vi "Engine(CSM).vi"(7 "Name(\"\" to use uuid)":string="TSEngine") -> ()   [LabVIEW 2020, in "CSMStand(Lite).lvlib"]
doc: "------------- lvcsm -------------\n[CSMStates]\nItem 0 = \"Idle\"\nItem 1 = \"CSM Documentation\"\nItem 2 = \"Error Handler\"\nItem 3 = \"VI Reference\"\nItem 4 = \"Critical Error\"\nItem 5 = \"Target Timeout Error\"\nItem 6 = \"Target Error\"\nItem 7 = \"Async Response\"\nItem 8 = \"Response\"\nItem 9 = \"Async Message Posted\"\nItem 10 = \"Initialize Core Data\"\nItem 11 = \"Exit\"\nItem 12 = \"Data: Initialize\"\nItem 13 = \"Data: Get Configuration\"\nItem 14 = \"Data: Get Internal Data\"\nItem 15 = \"Data: Set Configuration\"\nItem 16 = \"Data: Update Indicators\"\nItem 17 = \"Data: Cleanup\"\nItem 18 = \"Macro: Initialize\"\nItem 19 = \"Macro: Exit\"\nItem 20 = \"TS: Load Sequence\"\nItem 21 = \"TS: Unload Sequence\"\nItem 22 = \"TS: SinglePass\"\nItem 23 = \"TS: Terminate\"\n\n[CSMStatus]\nItem 0 = \"Error Occurred@Error Handler\"\nItem 1 = \"SequenceLoaded Event@TS: Load Sequence\"\nItem 2 = \"SequenceUnloaded Event@TS: Unload Sequence\""
uses:
  CSMStand(Lite).lvlib
  177df613-786b-4953-91e1-5a54b4498db6.vi
  e32ef8e6-06f2-447d-b550-f32965c6f747.vi
  42464f7e-1352-40b0-9025-febecf2bff56.vi
  28b741bb-94bb-4c2f-9535-6203235cad54.vi
  67be72c3-d4c2-4166-a53e-31f1adb5f8f9.vi
  <userlib>/_NEVSTOP/Communicable State Machine(CSM)/_Support/Common/Format Timestamp.vi
  <userlib>/_NEVSTOP/Communicable State Machine(CSM)/AdvanceAPI/CSM - Make String Arguments Safe.vi
  <userlib>/_NEVSTOP/Communicable State Machine(CSM)/AdvanceAPI/CSM - Break Down Multiple States String.vi
  <userlib>/_NEVSTOP/Communicable State Machine(CSM)/AdvanceAPI/CSM - Compact Multiple States.vi
  <userlib>/_NEVSTOP/Communicable State Machine(CSM)/AdvanceAPI/CSM - Keywords.vi
  <userlib>/_NEVSTOP/Communicable State Machine(CSM)/_Shared/Trim Single-line Text.vi
  <userlib>/_NEVSTOP/Communicable State Machine(CSM)/addons/API-String-Arugments-Support/_Support/Query Data as API String Arguments(variant).vi
  <userlib>/_NEVSTOP/Communicable State Machine(CSM)/addons/API-String-Arugments-Support/_Support/Convert API String Arguments to Data(variant).vi
  _Support/Working Thread.vi
  <userlib>/_NEVSTOP/Communicable State Machine(CSM)/AdvanceAPI/CSM - Get Module Attribute.vi
  <userlib>/_NEVSTOP/Communicable State Machine(CSM)/AdvanceAPI/CSM - Set Module Attribute.vi
  <userlib>/_NEVSTOP/Communicable State Machine(CSM)/Communicable State Machine.lvlib
  <userlib>/_NEVSTOP/Communicable State Machine(CSM)/addons/API-String-Arugments-Support/API String Arguments Support.lvlib
panel:
  out "State History":string
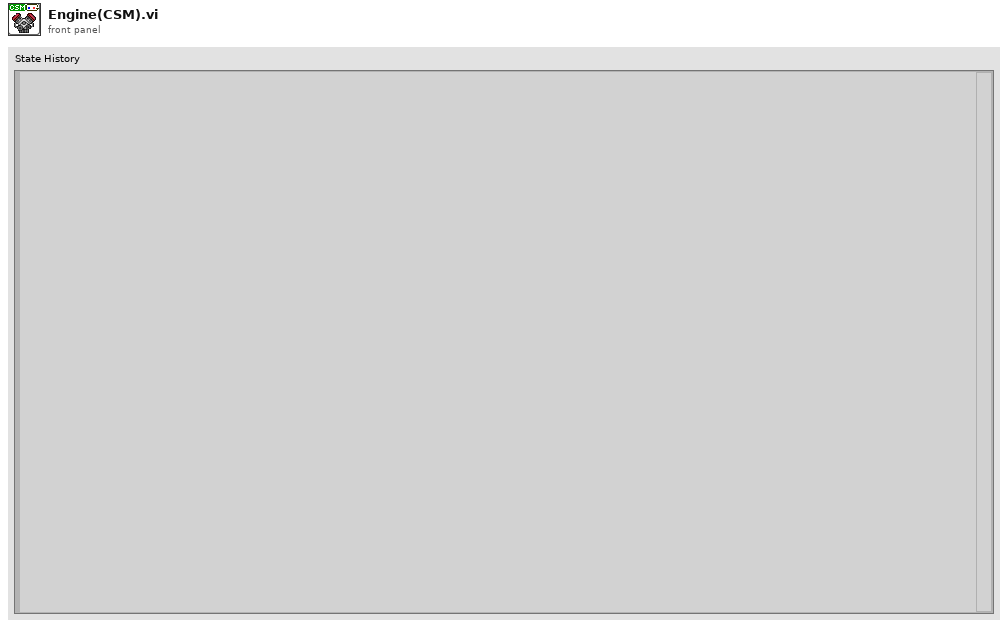
[diagram p1: front panel]
types:
  T1 = enum32{"Invalid", "Standard", "Closed", "Hidden", "Minimized", "Maximized"}
  T2 = enum32{"invalid app kind", "Development System", "Run Time System", "Student Edition", "Embedded LabVIEW", "Evaluation", "Custom"}
  T3 = typedef "Communicable State Machine.lvlib/_CSM_Response Source Message.ctl" = cluster{"‘State":string, "’Arguments":string, "’Error":errorcluster}
  T4 = cluster{"Current VI Reference":refnum<vi>, "Close Panel on Exit?":bool}
  T5 = cluster{"Core":cluster{"Current VI Reference":refnum<vi>, "Close Panel on Exit?":bool}, "Sequence":string}
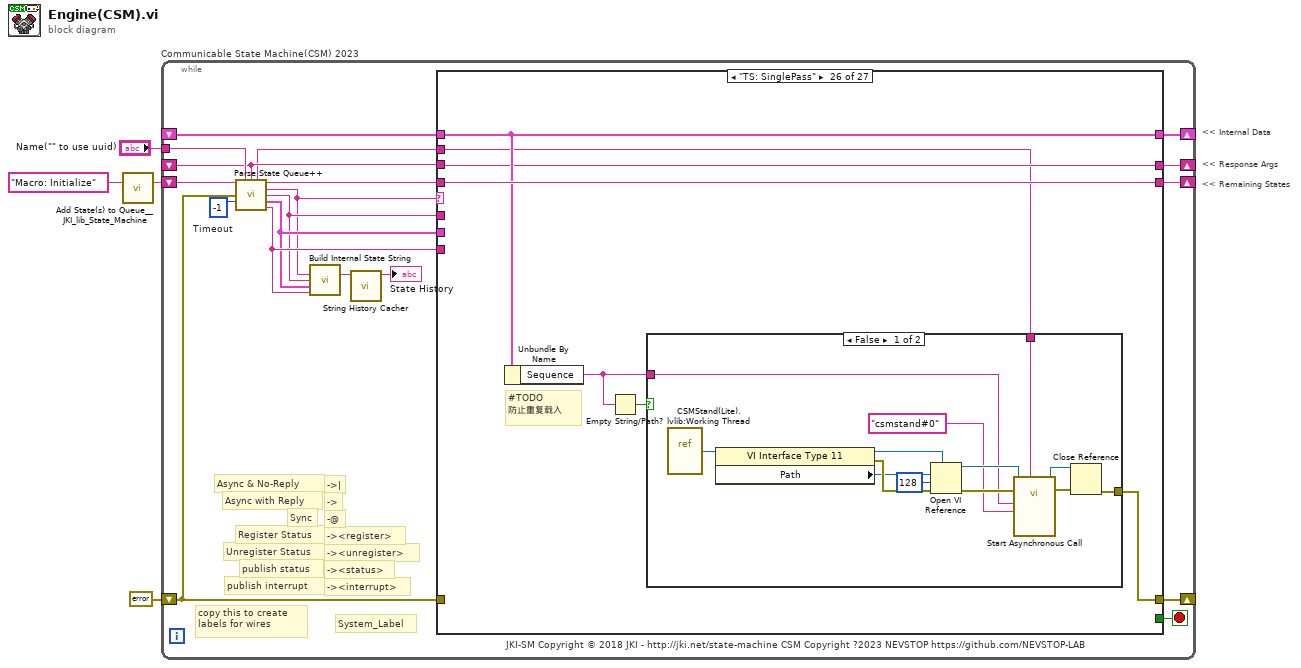
[diagram p0: block diagram]
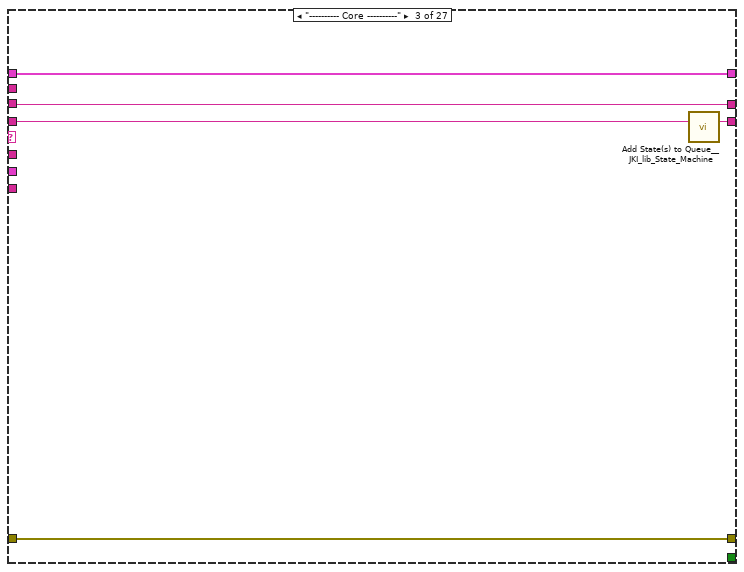
[diagram p4: hidden frame]
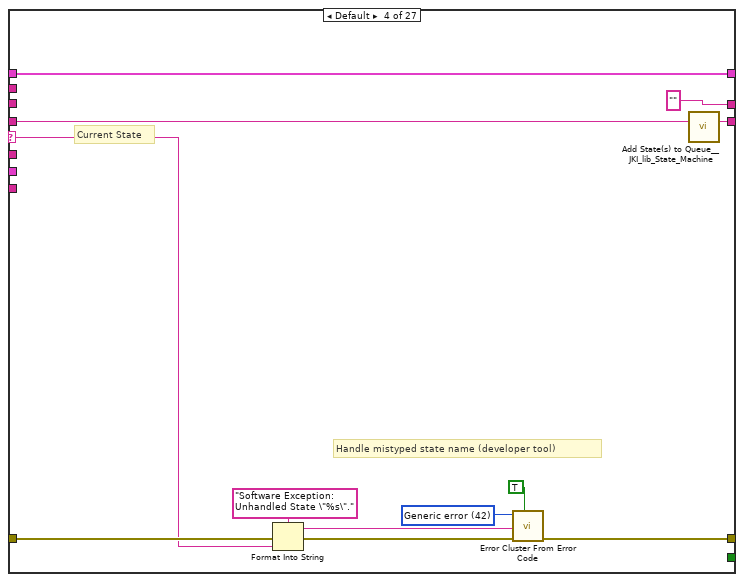
[diagram p5: hidden frame]
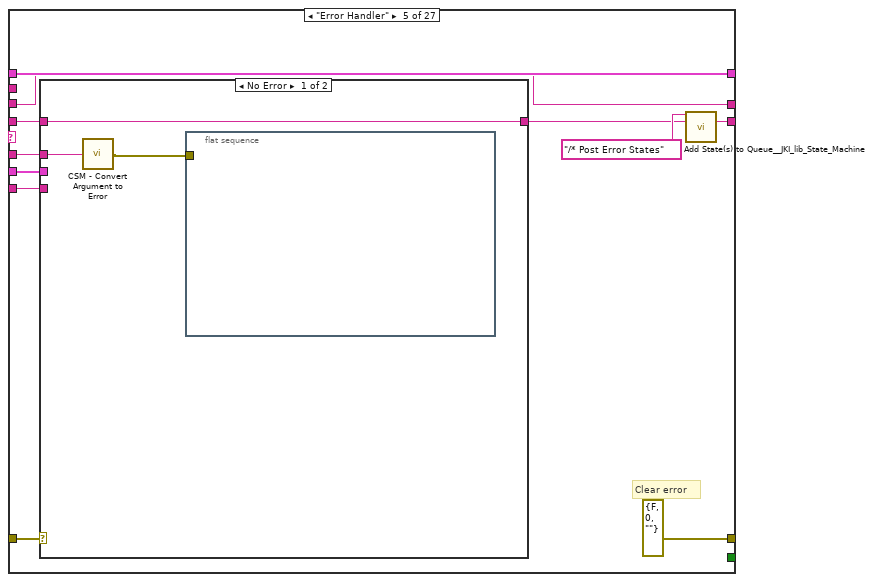
[diagram p6: hidden frame]
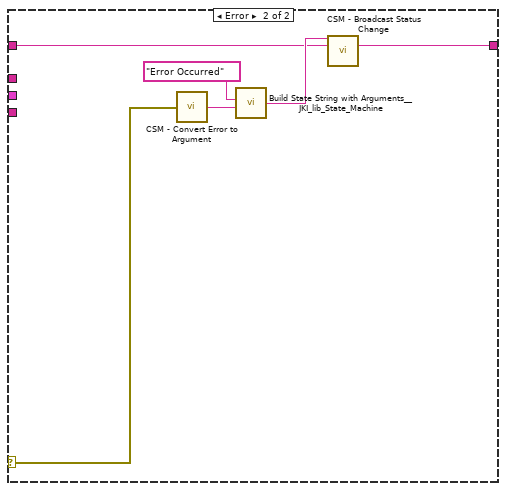
[diagram p7: hidden frame]
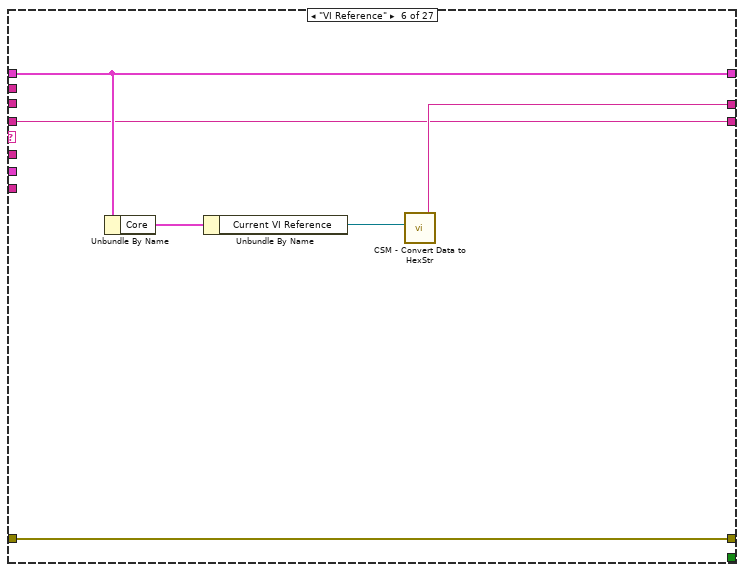
[diagram p8: hidden frame]
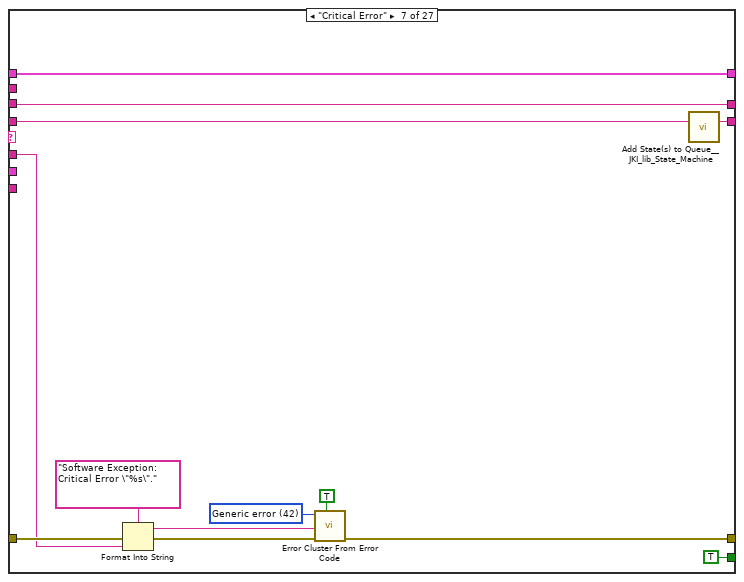
[diagram p9: hidden frame]
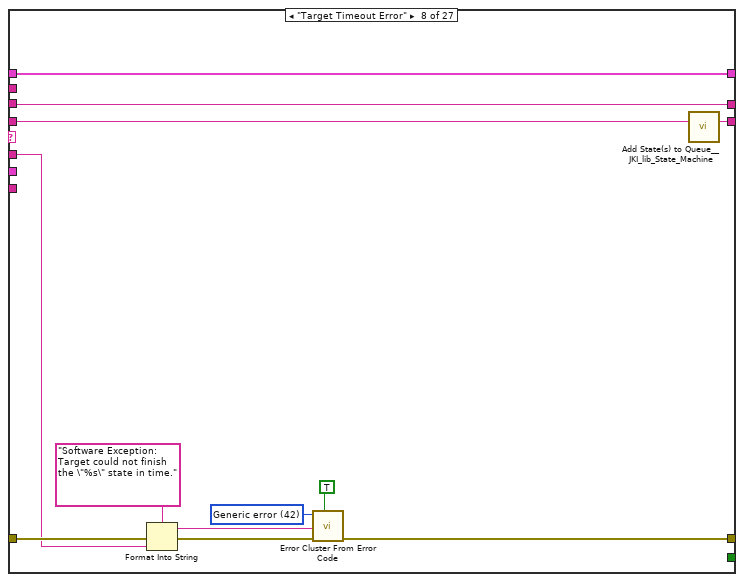
[diagram p10: hidden frame]
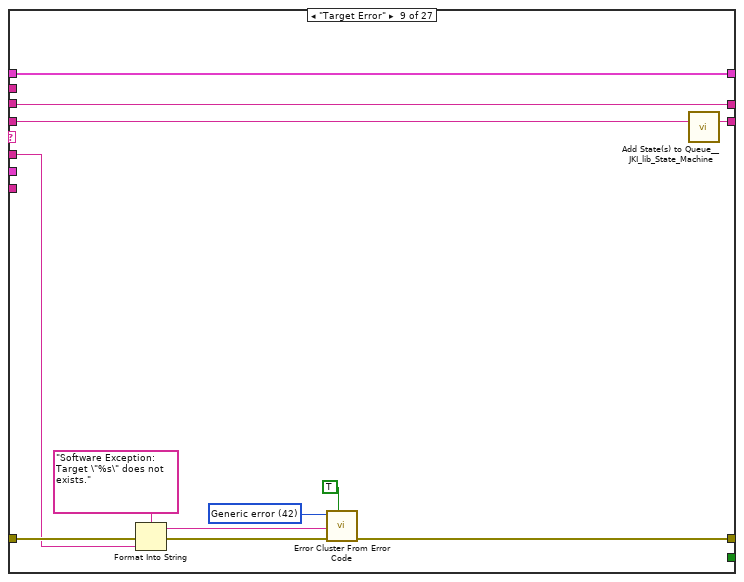
[diagram p11: hidden frame]
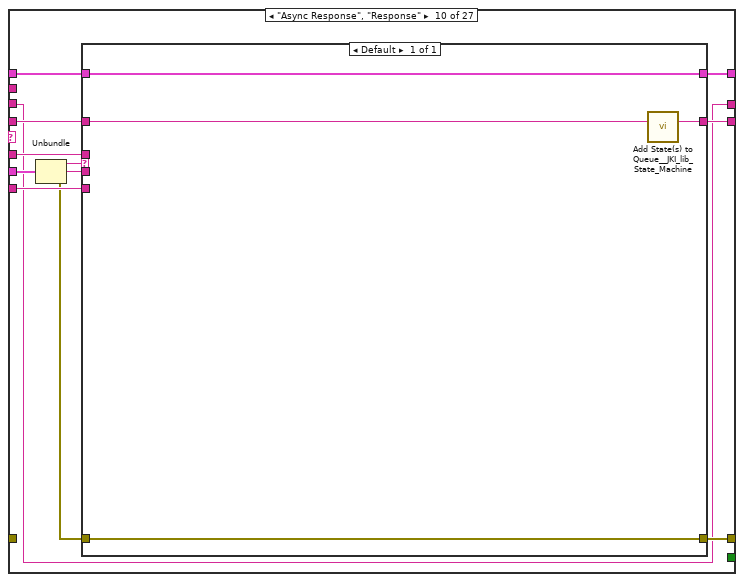
[diagram p12: hidden frame]
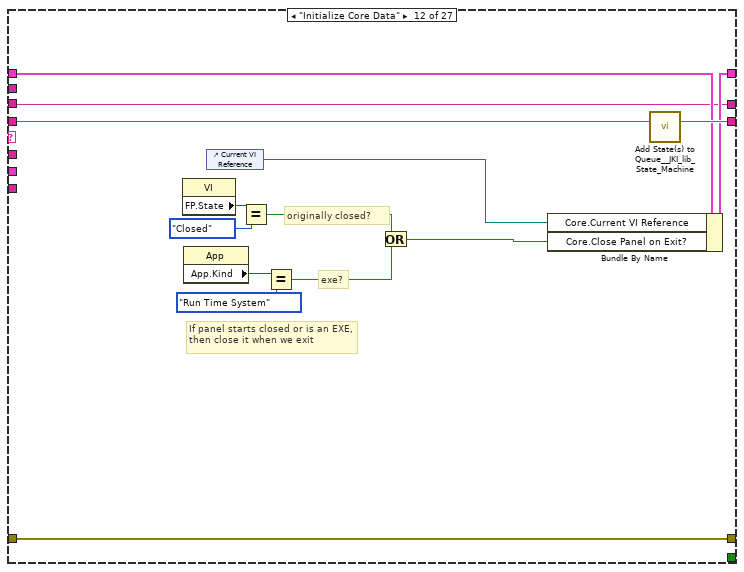
[diagram p14: hidden frame]
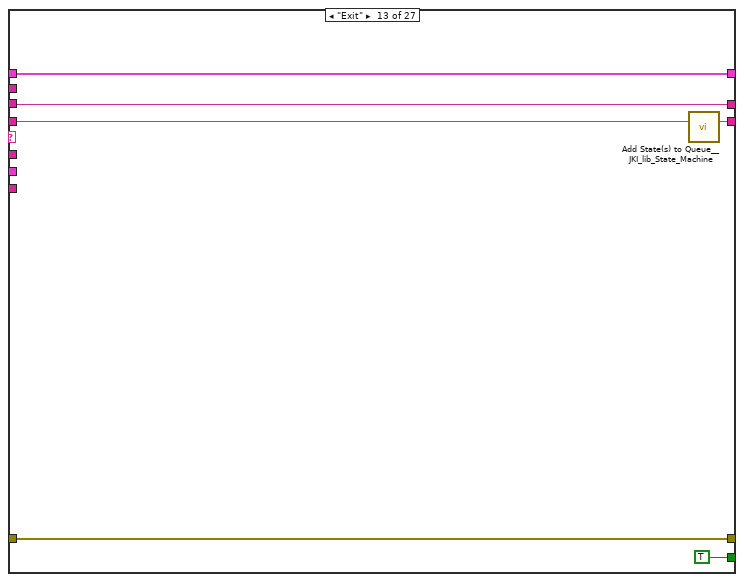
[diagram p15: hidden frame]
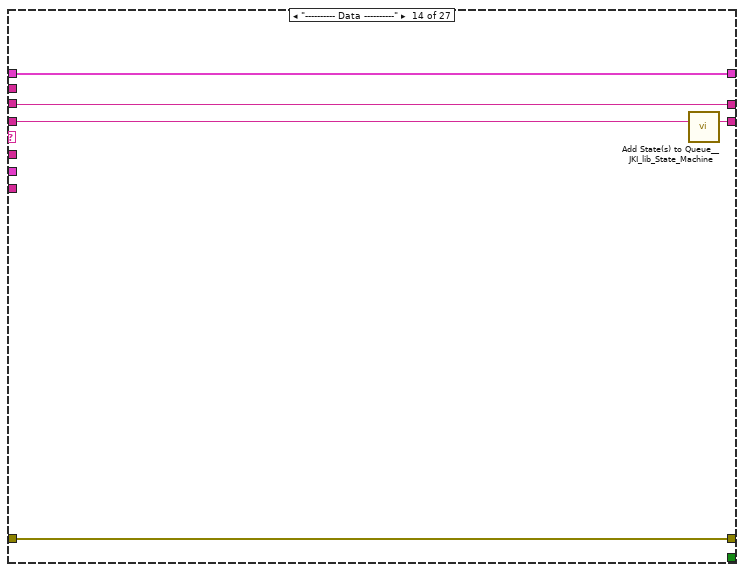
[diagram p16: hidden frame]
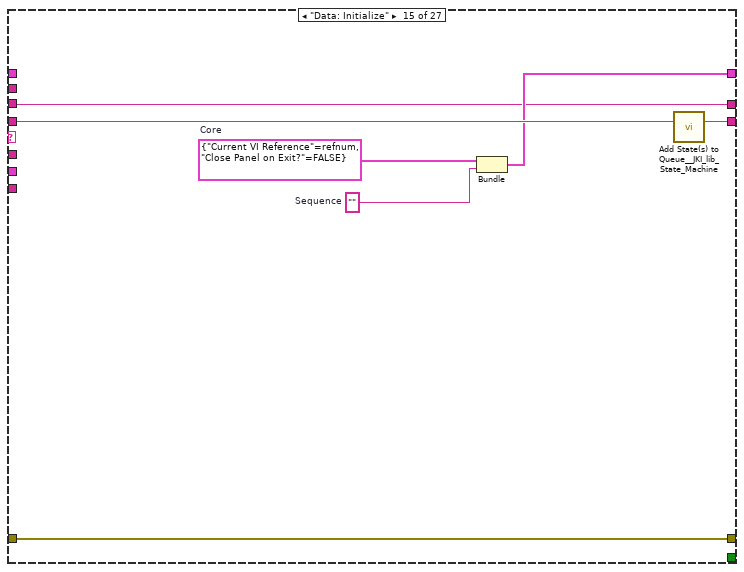
[diagram p17: hidden frame]
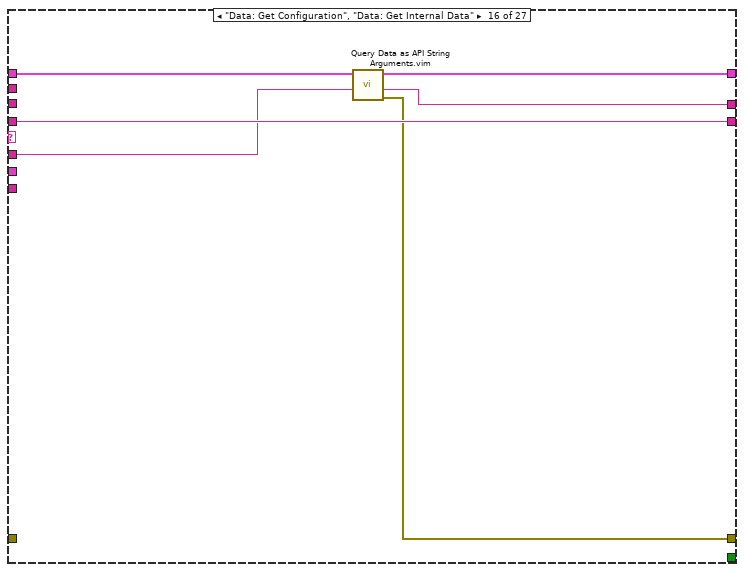
[diagram p18: hidden frame]
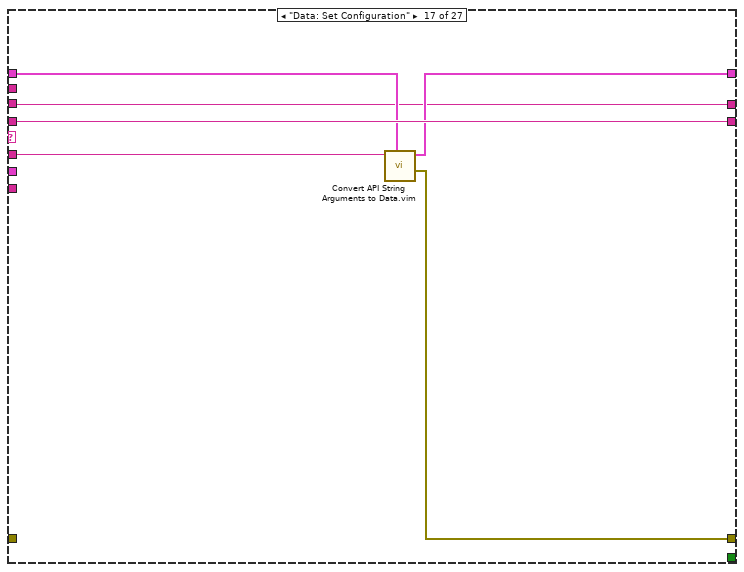
[diagram p19: hidden frame]
diagram:
  # "<< Internal Data"
  # "<< Response Args"
  # "<< Remaining States"
  n1 = call <vilib>:"Add State(s) to Queue__JKI_lib_State_Machine.vi"("State(s) in (\"\")"="Macro: Initialize" ("Init States(\"Macro: Initialize\")")) -> ("States Out"=w3:string)  [unwired: 14 in]
  n2 = while "Communicable State Machine(CSM) 2023" {
    shift-right: [w18] -> _
    shift-left: _ -> [w17]
    shift-right: [w21] -> _
    shift-left: errorcluster {"status"=FALSE, "code"=0, "source"=""} ("error out") -> [w5]
    shift-right: [w20] -> _
    shift-left: w3 -> [w22]
    tunnel: "Name(\"\" to use uuid)" -> [w14]
    shift-right: [w15] -> _
    shift-left: _ -> [w7]
    stop <- w19 stop-if-true
    w16 = -1  # Timeout
    # "copy this to create labels for wires"
    # "System_Label"
    # "-><interrupt>"
    # "-><status>"
    # "-><unregister>"
    # "-><register>"
    # "-@"
    # "->"
    # "->|"
    # "publish interrupt"
    # "publish status"
    # "Unregister Status"
    # "Register Status"
    # "Sync"
    # "Async with Reply"
    # "Async & No-Reply"
    # "JKI-SM Copyright © 2018 JKI - http://jki.net/state-machine CSM Copyright ?2023 NEVSTOP https://github.com/NEVSTOP-LAB"
    n3 = call <userlib>:"Parse State Queue++.vi"("State Queue"=w22, "Name (\"\" to Use UUID)"=w14, "Response Arguments"=w7, "Previous Error"=w5, "Dequeue (1 ms)"=w16) -> ("Name Used"=w6:string, "Remaining States"=w23:string, "Current State"=w8:string, "Arguments"=w9:string, ">> Response Source Message >>"=w10:T3, ">> Source CSM >>"=w11:string)  [unwired: 5 in]
    n4 = call <userlib>:"Build Internal State String.vi"("State"=w8, "Arguments (\"\")"=w9, ">> Response Source Message >>"=w10, "Source (\"\")"=w11) -> ("State With Arguments"=w12:string)  [unwired: 11 in]
    n5 = call <userlib>:"String History Cacher.vi"("String"=w12) -> ("String Cache"=→"State History":string)  [unwired: 10 in]
    n6 = case shown="\"TS: SinglePass\"" w8 {
      selector: w8 -> [_ _ _ w38 _ _ _ _ _ _ _ _ _ _ _ _ _ _ _ _ _ _ _ _ _ _ _]
      tunnel: w23 -> [w25 w30 w36 w42 w53 w70 w81 w94 w106 w117 w130 w145 w151 w156 w163 w169 w175 w178 w186 w191 w197 w203 w206 w213 w220 w230 w259]
      tunnel: w9 -> [_ _ _ _ w52 _ w77 w90 w102 w116 _ _ _ _ _ w164 w174 _ _ _ _ _ _ w209 _ _ w257]
      tunnel: w17 -> [w26 w29 w33 w40 w58 w74 w79 w92 w104 w118 w129 w138 w149 w153 _ w168 w173 w177 w181 w188 w194 w200 w205 w216 w222 w229 w258]
      tunnel: [w27 w31 w34 w44 errorcluster {"status"=FALSE, "code"=0, "source"=""} ("error out") w69 w83 w89 w101 w121 w131 w142 w148 w154 w160 w165 w171 w179 w182 w189 w195 w201 w207 w217 w223 w228 w251] -> w21
      tunnel: w5 -> [w27 w31 w34 w43 w56 w69 w82 w95 w107 _ w131 w142 w148 w154 w160 _ _ w179 w183 w189 w195 w201 w207 w217 w223 _ _]
      tunnel: [w25 w30 w35 w41 w54 w70 w80 w93 w105 w119 w130 w144 w150 w155 w162 w169 w175 w178 w185 w190 w196 w202 w206 w214 w221 w230 w259] -> w20
      tunnel: [_ _ _ _ _ _ TRUE _ _ _ _ _ TRUE _ _ _ _ _ _ _ _ _ _ _ _ _ _] -> w19
      tunnel: [w26 w29 w33 w40 w58 w74 w79 w92 w104 w120 w129 w143 w149 w153 w161 w167 w172 w177 w181 w188 w194 w200 w205 w215 w222 w229 w258] -> w18
      tunnel: w11 -> [_ _ _ _ w51 _ _ _ _ w114 _ _ _ _ _ _ _ _ _ _ _ _ _ _ _ _ _]
      tunnel: w10 -> [_ _ _ _ w50 _ _ _ _ w115 _ _ _ _ _ _ _ _ _ _ _ _ _ _ _ _ _]
      tunnel: [w24 w28 w32 "" w49 w71 w75 w88 w100 w112 w128 w132 w146 w152 w157 w166 w170 w176 w180 w187 w192 w198 w204 w208 w218 w227 w253] -> w15
      tunnel: w6 -> [_ _ _ _ _ _ _ _ _ _ _ _ _ _ _ _ _ _ _ _ _ _ _ _ _ w226 w247]
      tunnel: w7 -> [w24 w28 w32 _ w49 _ w75 w88 w100 w112 w128 w132 w146 w152 w157 _ w170 w176 w180 w187 w192 w198 w204 w208 w218 w227 w253]
      frame "", "Idle" {
      }
      frame "CSM Documentation" {
      }
      frame "---------- Core ----------" {
        n7 = call <vilib>:"Add State(s) to Queue__JKI_lib_State_Machine.vi"("State(s) in (\"\")"=w36) -> ("States Out"=w35:string)  [unwired: 14 in]
      }
      frame Default {
        w47 = 42 items=["No error", "Argument error", "Memory is full", "Out of zone", "End of file", "File already open", "Generic file I/O error", "File not found", "File permission error", "Disk is full", "Duplicate path", "Too many files open", "System feature not enabled", "Resource file not found", "Cannot add resource", "Resource not found", "Image not found", "Image memory error", "Pen does not exist", "Config type invalid", "Config token not found", "Config parse error", "Config memory error", "Bad external code format", "Bad external code offset", "External code not present", "Null window", "Destroy window error", "Null menu", "Print aborted", "Bad print record", "Print driver error", "Windows error during printing", "Memory error during printing", "Print dialog error", "Generic print error", "Invalid device refnum", "Device not found", "Device parameter error", "Device unit error", "Cannot open device", "Device call aborted", "Generic error", "Cancelled by user", "Object ID too low", "Object ID too high", "Object not in heap", "Unknown heap", "Unknown object (invalid DefProc)", "Unknown object (DefProc not in table)", "Message out of range", "Invalid (null) method", "Unknown message", "Manager call not supported", "Bad address", "Network operation in progress", "Network operation timed out", "Connection is busy", "Network attribute not supported", "Network error", "Address in use", "System out of memory", "Connection aborted", "Connection refused", "Not connected", "Already connected", "Connection closed", "Initialization error (interapplication manager)", "Bad occurrence", "Wait on unbound occurrence handler", "Occurrence queue overflow", "Datalog type conflict", "Unused", "Unrecognized type (interapplication manager)", "Memory corrupt", "Failed to make temporary DLL", "Old CIN version", "Drag socket not found", "Failed to load drop-object", "Failed to register OLE object", "Failed to release OLE object", "Format specifier type mismatch", "Unknown format specifier", "Too few format specifiers", "Too many format specifiers", "Scan failed", "Newer CIN version", "Error converting to variant", "Runtime menu error", "Password tampered", "Variant attribute not found", "Incompatible variant data type", "Event data is not available", "Event Store is not present", "Occurrence is not found", "Event Queue is not created", "Event info is not available", "Refnum passed is NULL", "Error retrieving Class GUID", "Error retrieving CoClass GUID", "Error retrieving TypeLib GUID.", "Bad built application magic bytes.", "Specific driver is different from the specific driver associated with the Logical Name.", "There is no session opened to the class driver.", "Max Error", "MAX - Error with config objects", "MAX - Error loading configuration", "MAX - Group not supported"]
        # "Current State"
        # "Handle mistyped state name (developer tool)"
        n8 = Format Into String(format string="Software Exception: Unhandled State \"%s\"." ("message"), error in=w43, w38) -> (resulting string=w46:string, error out=w45:errorcluster)  [unwired: 1 in]
        n9 = call <vilib>:"Error Cluster From Error Code.vi"("show call chain? (False)"=TRUE, "error in (no error)"=w45, "error message (\"\")"=w46, "error code (0)"=w47) -> ("error out"=w44:errorcluster)  [unwired: 5 in]
        n10 = call <vilib>:"Add State(s) to Queue__JKI_lib_State_Machine.vi"("State(s) in (\"\")"=w42) -> ("States Out"=w41:string)  [unwired: 14 in]
      }
      frame "Error Handler" {
        # "Clear error"
        n11 = case shown="No Error" w56 {
          selector: w56 -> [_ w63]
          tunnel: [w62 w65] -> w55
          tunnel: w53 -> [w62 w64]
          tunnel: w52 -> [w61 _]
          tunnel: w51 -> [_ _]
          tunnel: w50 -> [_ _]
          frame No Error {
            n12 = call <userlib>:"CSM - Convert Argument to Error.vi"("Argument"=w61) -> ("Error"=w60:errorcluster)  [unwired: 4 in]
            n13 = flat-sequence {
              tunnel: w60 -> [_]
              frame #0 {
              }
            }
          }
          frame Error {
            n14 = call <userlib>:"CSM - Convert Error to Argument.vi"("Error"=w63) -> ("Argument"=w67:string)  [unwired: 4 in]
            n15 = call <vilib>:"Build State String with Arguments__JKI_lib_State_Machine.vi"("Arguments (\"\")"=w67, "State"="Error Occurred" ("Status with Arguments")) -> ("State with Arguments"=w66:string)  [unwired: 4 in]
            n16 = call <userlib>:"CSM - Broadcast Status Change.vi"("Status With Arguments"=w66, "State Queue"=w64) -> ("Remaining States"=w65:string)  [unwired: 13 in]
          }
        }
        n17 = call <vilib>:"Add State(s) to Queue__JKI_lib_State_Machine.vi"("State(s) in Front (\"\")"="/* Post Error States", "State(s) in (\"\")"=w55) -> ("States Out"=w54:string)  [unwired: 13 in]
      }
      frame "VI Reference" {
        n18 = Unbundle By Name(w74) -> ("Core"=w73:T4)
        n19 = Unbundle By Name(w73) -> ("Current VI Reference"=w72:refnum<vi>)
        n20 = call <userlib>:"CSM - Convert Data to HexStr.vi"("Variant"=w72) -> ("HEX String (0-9,A-F)"=w71:string)  [unwired: 8 in]
      }
      frame "Critical Error" {
        w86 = 42 items=["No error", "Argument error", "Memory is full", "Out of zone", "End of file", "File already open", "Generic file I/O error", "File not found", "File permission error", "Disk is full", "Duplicate path", "Too many files open", "System feature not enabled", "Resource file not found", "Cannot add resource", "Resource not found", "Image not found", "Image memory error", "Pen does not exist", "Config type invalid", "Config token not found", "Config parse error", "Config memory error", "Bad external code format", "Bad external code offset", "External code not present", "Null window", "Destroy window error", "Null menu", "Print aborted", "Bad print record", "Print driver error", "Windows error during printing", "Memory error during printing", "Print dialog error", "Generic print error", "Invalid device refnum", "Device not found", "Device parameter error", "Device unit error", "Cannot open device", "Device call aborted", "Generic error", "Cancelled by user", "Object ID too low", "Object ID too high", "Object not in heap", "Unknown heap", "Unknown object (invalid DefProc)", "Unknown object (DefProc not in table)", "Message out of range", "Invalid (null) method", "Unknown message", "Manager call not supported", "Bad address", "Network operation in progress", "Network operation timed out", "Connection is busy", "Network attribute not supported", "Network error", "Address in use", "System out of memory", "Connection aborted", "Connection refused", "Not connected", "Already connected", "Connection closed", "Initialization error (interapplication manager)", "Bad occurrence", "Wait on unbound occurrence handler", "Occurrence queue overflow", "Datalog type conflict", "Unused", "Unrecognized type (interapplication manager)", "Memory corrupt", "Failed to make temporary DLL", "Old CIN version", "Drag socket not found", "Failed to load drop-object", "Failed to register OLE object", "Failed to release OLE object", "Format specifier type mismatch", "Unknown format specifier", "Too few format specifiers", "Too many format specifiers", "Scan failed", "Newer CIN version", "Error converting to variant", "Runtime menu error", "Password tampered", "Variant attribute not found", "Incompatible variant data type", "Event data is not available", "Event Store is not present", "Occurrence is not found", "Event Queue is not created", "Event info is not available", "Refnum passed is NULL", "Error retrieving Class GUID", "Error retrieving CoClass GUID", "Error retrieving TypeLib GUID.", "Bad built application magic bytes.", "Specific driver is different from the specific driver associated with the Logical Name.", "There is no session opened to the class driver.", "Max Error", "MAX - Error with config objects", "MAX - Error loading configuration", "MAX - Group not supported"]
        n21 = Format Into String(format string="Software Exception: Critical Error \"%s\"." ("message"), error in=w82, w77) -> (resulting string=w85:string, error out=w84:errorcluster)  [unwired: 1 in]
        n22 = call <vilib>:"Error Cluster From Error Code.vi"("show call chain? (False)"=TRUE, "error in (no error)"=w84, "error message (\"\")"=w85, "error code (0)"=w86) -> ("error out"=w83:errorcluster)  [unwired: 5 in]
        n23 = call <vilib>:"Add State(s) to Queue__JKI_lib_State_Machine.vi"("State(s) in (\"\")"=w81) -> ("States Out"=w80:string)  [unwired: 14 in]
      }
      frame "Target Timeout Error" {
        w98 = 42 items=["No error", "Argument error", "Memory is full", "Out of zone", "End of file", "File already open", "Generic file I/O error", "File not found", "File permission error", "Disk is full", "Duplicate path", "Too many files open", "System feature not enabled", "Resource file not found", "Cannot add resource", "Resource not found", "Image not found", "Image memory error", "Pen does not exist", "Config type invalid", "Config token not found", "Config parse error", "Config memory error", "Bad external code format", "Bad external code offset", "External code not present", "Null window", "Destroy window error", "Null menu", "Print aborted", "Bad print record", "Print driver error", "Windows error during printing", "Memory error during printing", "Print dialog error", "Generic print error", "Invalid device refnum", "Device not found", "Device parameter error", "Device unit error", "Cannot open device", "Device call aborted", "Generic error", "Cancelled by user", "Object ID too low", "Object ID too high", "Object not in heap", "Unknown heap", "Unknown object (invalid DefProc)", "Unknown object (DefProc not in table)", "Message out of range", "Invalid (null) method", "Unknown message", "Manager call not supported", "Bad address", "Network operation in progress", "Network operation timed out", "Connection is busy", "Network attribute not supported", "Network error", "Address in use", "System out of memory", "Connection aborted", "Connection refused", "Not connected", "Already connected", "Connection closed", "Initialization error (interapplication manager)", "Bad occurrence", "Wait on unbound occurrence handler", "Occurrence queue overflow", "Datalog type conflict", "Unused", "Unrecognized type (interapplication manager)", "Memory corrupt", "Failed to make temporary DLL", "Old CIN version", "Drag socket not found", "Failed to load drop-object", "Failed to register OLE object", "Failed to release OLE object", "Format specifier type mismatch", "Unknown format specifier", "Too few format specifiers", "Too many format specifiers", "Scan failed", "Newer CIN version", "Error converting to variant", "Runtime menu error", "Password tampered", "Variant attribute not found", "Incompatible variant data type", "Event data is not available", "Event Store is not present", "Occurrence is not found", "Event Queue is not created", "Event info is not available", "Refnum passed is NULL", "Error retrieving Class GUID", "Error retrieving CoClass GUID", "Error retrieving TypeLib GUID.", "Bad built application magic bytes.", "Specific driver is different from the specific driver associated with the Logical Name.", "There is no session opened to the class driver.", "Max Error", "MAX - Error with config objects", "MAX - Error loading configuration", "MAX - Group not supported"]
        n24 = Format Into String(format string="Software Exception: Target could not finish the \"%s\" state in time." ("message"), error in=w95, w90) -> (resulting string=w97:string, error out=w96:errorcluster)  [unwired: 1 in]
        n25 = call <vilib>:"Error Cluster From Error Code.vi"("show call chain? (False)"=TRUE, "error in (no error)"=w96, "error message (\"\")"=w97, "error code (0)"=w98) -> ("error out"=w89:errorcluster)  [unwired: 5 in]
        n26 = call <vilib>:"Add State(s) to Queue__JKI_lib_State_Machine.vi"("State(s) in (\"\")"=w94) -> ("States Out"=w93:string)  [unwired: 14 in]
      }
      frame "Target Error" {
        w110 = 42 items=["No error", "Argument error", "Memory is full", "Out of zone", "End of file", "File already open", "Generic file I/O error", "File not found", "File permission error", "Disk is full", "Duplicate path", "Too many files open", "System feature not enabled", "Resource file not found", "Cannot add resource", "Resource not found", "Image not found", "Image memory error", "Pen does not exist", "Config type invalid", "Config token not found", "Config parse error", "Config memory error", "Bad external code format", "Bad external code offset", "External code not present", "Null window", "Destroy window error", "Null menu", "Print aborted", "Bad print record", "Print driver error", "Windows error during printing", "Memory error during printing", "Print dialog error", "Generic print error", "Invalid device refnum", "Device not found", "Device parameter error", "Device unit error", "Cannot open device", "Device call aborted", "Generic error", "Cancelled by user", "Object ID too low", "Object ID too high", "Object not in heap", "Unknown heap", "Unknown object (invalid DefProc)", "Unknown object (DefProc not in table)", "Message out of range", "Invalid (null) method", "Unknown message", "Manager call not supported", "Bad address", "Network operation in progress", "Network operation timed out", "Connection is busy", "Network attribute not supported", "Network error", "Address in use", "System out of memory", "Connection aborted", "Connection refused", "Not connected", "Already connected", "Connection closed", "Initialization error (interapplication manager)", "Bad occurrence", "Wait on unbound occurrence handler", "Occurrence queue overflow", "Datalog type conflict", "Unused", "Unrecognized type (interapplication manager)", "Memory corrupt", "Failed to make temporary DLL", "Old CIN version", "Drag socket not found", "Failed to load drop-object", "Failed to register OLE object", "Failed to release OLE object", "Format specifier type mismatch", "Unknown format specifier", "Too few format specifiers", "Too many format specifiers", "Scan failed", "Newer CIN version", "Error converting to variant", "Runtime menu error", "Password tampered", "Variant attribute not found", "Incompatible variant data type", "Event data is not available", "Event Store is not present", "Occurrence is not found", "Event Queue is not created", "Event info is not available", "Refnum passed is NULL", "Error retrieving Class GUID", "Error retrieving CoClass GUID", "Error retrieving TypeLib GUID.", "Bad built application magic bytes.", "Specific driver is different from the specific driver associated with the Logical Name.", "There is no session opened to the class driver.", "Max Error", "MAX - Error with config objects", "MAX - Error loading configuration", "MAX - Group not supported"]
        n27 = Format Into String(format string="Software Exception: Target \"%s\" does not exists." ("message"), error in=w107, w102) -> (resulting string=w109:string, error out=w108:errorcluster)  [unwired: 1 in]
        n28 = call <vilib>:"Error Cluster From Error Code.vi"("show call chain? (False)"=TRUE, "error in (no error)"=w108, "error message (\"\")"=w109, "error code (0)"=w110) -> ("error out"=w101:errorcluster)  [unwired: 5 in]
        n29 = call <vilib>:"Add State(s) to Queue__JKI_lib_State_Machine.vi"("State(s) in (\"\")"=w106) -> ("States Out"=w105:string)  [unwired: 14 in]
      }
      frame "Async Response", "Response" {
        n30 = Unbundle(w115) -> ("‘State"=w123:string, "’Arguments"=w122:string, "’Error"=w113:errorcluster)
        n31 = case shown="Default" w123 {
          tunnel: [w124] -> w119
          tunnel: w117 -> [w125]
          tunnel: [w127] -> w120
          tunnel: w118 -> [w127]
          tunnel: [w126] -> w121
          tunnel: w113 -> [w126]
          tunnel: w114 -> [_]
          tunnel: w116 -> [_]
          tunnel: w122 -> [_]
          frame Default {
            n32 = call <vilib>:"Add State(s) to Queue__JKI_lib_State_Machine.vi"("State(s) in (\"\")"=w125) -> ("States Out"=w124:string)  [unwired: 14 in]
          }
        }
      }
      frame "Async Message Posted" {
      }
      frame "Initialize Core Data" {
        # "originally closed?"
        # "exe?"
        # "If panel starts closed or is an EXE, then close it when we exit"
        n33 = property class="VI"() -> ("FP.State"=w135:T1)  [unwired: 2 in, 2 out]
        n34 = property class="App"() -> ("App.Kind"=w141:T2)  [unwired: 2 in, 2 out]
        n35 = control-ref of="Current VI Reference"() -> (w136:refnum<vi>)
        n36 = Equal?(x=w135, y=T1."Closed" ("Front Panel Window:State")) -> (x = y?=w133:bool)
        n37 = Equal?(x=w141, y=T2."Run Time System" ("Application:Kind")) -> (x = y?=w139:bool)
        n38 = Or(x=w133, y=w139) -> (x .or. y?=w137:bool)
        n39 = Bundle By Name(cluster=w138, "Core.Current VI Reference"=w136, "Core.Close Panel on Exit?"=w137) -> (w143:T5)
        n40 = call <vilib>:"Add State(s) to Queue__JKI_lib_State_Machine.vi"("State(s) in (\"\")"=w145) -> ("States Out"=w144:string)  [unwired: 14 in]
      }
      frame "Exit" {
        n41 = call <vilib>:"Add State(s) to Queue__JKI_lib_State_Machine.vi"("State(s) in (\"\")"=w151) -> ("States Out"=w150:string)  [unwired: 14 in]
      }
      frame "---------- Data ----------" {
        n42 = call <vilib>:"Add State(s) to Queue__JKI_lib_State_Machine.vi"("State(s) in (\"\")"=w156) -> ("States Out"=w155:string)  [unwired: 14 in]
      }
      frame "Data: Initialize" {
        w158 = ""  # Sequence
        w159 = T4 {"Current VI Reference"=refnum, "Close Panel on Exit?"=FALSE}  # Core
        n43 = Bundle("Core"=w159, "Sequence"=w158) -> (w161:T5)  [unwired: 1 in]
        n44 = call <vilib>:"Add State(s) to Queue__JKI_lib_State_Machine.vi"("State(s) in (\"\")"=w163) -> ("States Out"=w162:string)  [unwired: 14 in]
      }
      frame "Data: Get Configuration", "Data: Get Internal Data" {
        n45 = call "Query Data as API String Arguments.vim"("Setting Name"=w164, "Internal Data"=w168) -> ("error"=w165:errorcluster, "Setting as String"=w166:string, "Internal Data(dup)"=w167:T5)  [unwired: 7 in]
      }
      frame "Data: Set Configuration" {
        n46 = call "Convert API String Arguments to Data.vim"("Type"=w173, "String"=w174) -> ("error"=w171:errorcluster, "Data"=w172:T5)  [unwired: 6 in]
      }
      frame "Data: Update Indicators" {
      }
      frame "Data: Cleanup" {
        n47 = Unbundle By Name(w181) -> ("Core.Current VI Reference"=w184:refnum<vi>)
        n48 = Close Reference(reference=w184, error in (no error)=w183) -> (error out=w182:errorcluster)
        n49 = call <vilib>:"Add State(s) to Queue__JKI_lib_State_Machine.vi"("State(s) in (\"\")"=w186) -> ("States Out"=w185:string)  [unwired: 14 in]
      }
      frame "---------- Macro ----------" {
        n50 = call <vilib>:"Add State(s) to Queue__JKI_lib_State_Machine.vi"("State(s) in (\"\")"=w191) -> ("States Out"=w190:string)  [unwired: 14 in]
      }
      frame "Macro: Initialize" {
        n51 = call <vilib>:"Add State(s) to Queue__JKI_lib_State_Machine.vi"("State(s) in Front (\"\")"="Data: Initialize\nInitialize Core Data\nData: Update Indicators", "State(s) in (\"\")"=w197) -> ("States Out"=w196:string)  [unwired: 13 in]
      }
      frame "Macro: Exit" {
        n52 = call <vilib>:"Add State(s) to Queue__JKI_lib_State_Machine.vi"("State(s) in Front (\"\")"="Data: Cleanup\nExit", "State(s) in (\"\")"=w203) -> ("States Out"=w202:string)  [unwired: 13 in]
      }
      frame "---------- TestStand API ----------" {
      }
      frame "TS: Load Sequence" {
        n53 = call <userlib>:"CSM - Revert Arguments-Safe String.vi"("Safe Argument String"=w209) -> ("Origin Argument String"=w210:string)  [unwired: 8 in]
        n54 = Bundle By Name(cluster=w216, "Sequence"=w210) -> (w215:T5)
        n55 = call <vilib>:"Build State String with Arguments__JKI_lib_State_Machine.vi"("Arguments (\"\")"=w209, "State"="SequenceLoaded Event" ("Status with Arguments")) -> ("State with Arguments"=w212:string)  [unwired: 4 in]
        n56 = call <userlib>:"CSM - Broadcast Status Change.vi"("Status With Arguments"=w212, "State Queue"=w213) -> ("Remaining States"=w214:string)  [unwired: 13 in]
      }
      frame "TS: Unload Sequence" {
        n57 = call <userlib>:"CSM - Broadcast Status Change.vi"("Status With Arguments"="SequenceUnloaded Event" ("Status with Arguments"), "State Queue"=w220) -> ("Remaining States"=w221:string)  [unwired: 13 in]
      }
      frame "TS: SinglePass" {
        # "#TODO\n防止重复载入"
        n58 = Unbundle By Name(w229) -> ("Sequence"=w225:string)
        n59 = Empty String/Path?(string/path=w225) -> (empty?=w224:bool)
        n60 = case shown="False" w224 {
          tunnel: [w234 _] -> w228
          tunnel: w226 -> [w233 _]
          tunnel: w225 -> [w231 _]
          frame False {
            n61 = vi-ref "CSMStand(Lite).lvlib:Working Thread.vi"() -> (w236:refnum<vi>)
            n62 = property class="VI Interface Type 11"(reference=w236) -> (reference out=w240:refnum<vi>, error out=w238:errorcluster, "Path"=w237:path)  [unwired: 1 in]
            n63 = Open VI Reference(type specifier VI Refnum (for type only)=w240, vi path=w237, options=128, error in (no error)=w238) -> (vi reference=w239:refnum<vi>, error out=w235:errorcluster)  [unwired: 2 in]
            n64 = call-by-ref "Start Asynchronous Call"(reference=w239, error in=w235, "EngineCSM"=w233, "socketIndex"="csmstand#0" ("Thread#"), "Sequence"=w231) -> (reference out=w242:refnum<vi>, error out=w241:errorcluster)  [unwired: 9 in]
            n65 = Close Reference(reference=w242, error in (no error)=w241) -> (error out=w234:errorcluster)
          }
          frame True {
          }
        }
      }
      frame "TS: Terminate" {
        w255 = "csmstand#0" ("Thread#")
        (unwired) "Terminated by CSMStand" ("reason(\"\")")
        # "Engine is using this to Stop"
        n66 = call "Convert API String Arguments to Data.vim"("Type"=w255, "String"=w257) -> ("error"=w252:errorcluster, "Data"=w254:string)  [unwired: 6 in]
        n67 = Empty String/Path?(string/path=w254) -> (empty?=w256:bool)
        n68 = Select(t=w255, s=w256, f=w254) -> (s? t:f=w249:string)
        n69 = call <userlib>:"Concatenate Strings If not Empty_csm.vi"("String"=w249, "seperator(:)"="#", "prefix"=w247) -> ("result"=w245:string)  [unwired: 2 in]
        n70 = call "CSM Get Module Attribute.vim"("CSM Name"=w247, "Attribute"=w245, "Error In"=w252) -> ("CSM Name (Dup)"=w246:string, "Found"=w244:bool, "error out"=w248:errorcluster)  [unwired: 8 in, 2 out]
        n71 = case shown="True" w244 {
          tunnel: [w260 w265] -> w251
          tunnel: w248 -> [w260 w264]
          tunnel: w246 -> [_ w263]
          tunnel: w245 -> [_ w262]
          frame False {
          }
          frame True {
            n72 = call "CSM Set Module Attribute.vim"("CSM Name"=w263, "Attribute"=w262, "Value"=TRUE, "Error In"=w264) -> ("error out"=w265:errorcluster)  [unwired: 8 in, 3 out]
          }
        }
      }
    }
  }
